vi "Set Value (U32).vi"(8 "error in":errorcluster, 9 "Value":u32, 10 "TPCANParameter":T2, 11 "TPCANHandle in":T1 items=["PCAN_NONEBUS"=0, "PCAN_USBBUS1"=81, "PCAN_USBBUS2"=82, "PCAN_USBBUS3"=83, "PCAN_USBBUS4"=84, "PCAN_USBBUS5"=85, "PCAN_USBBUS6"=86, "PCAN_USBBUS7"=87, "PCAN_USBBUS8"=88, "PCAN_USBBUS9"=1289, "PCAN_USBBUS10"=1290, "PCAN_USBBUS11"=1291, "PCAN_USBBUS12"=1292, "PCAN_USBBUS13"=1293, "PCAN_USBBUS14"=1294, "PCAN_USBBUS15"=1295, "PCAN_USBBUS16"=1296]) -> (0 "error out":errorcluster, 3 "TPCANHandle out":T1 items=["PCAN_NONEBUS"=0, "PCAN_USBBUS1"=81, "PCAN_USBBUS2"=82, "PCAN_USBBUS3"=83, "PCAN_USBBUS4"=84, "PCAN_USBBUS5"=85, "PCAN_USBBUS6"=86, "PCAN_USBBUS7"=87, "PCAN_USBBUS8"=88, "PCAN_USBBUS9"=1289, "PCAN_USBBUS10"=1290, "PCAN_USBBUS11"=1291, "PCAN_USBBUS12"=1292, "PCAN_USBBUS13"=1293, "PCAN_USBBUS14"=1294, "PCAN_USBBUS15"=1295, "PCAN_USBBUS16"=1296], 5 "TPCANStatus":u32)   [LabVIEW 2020, in "PCANBasic.lvlib"]
uses:
  PCANBasic.lvlib
  peak/PCANBasic64.dll
  TPCANParameter.ctl
  TPCANHandle.ctl
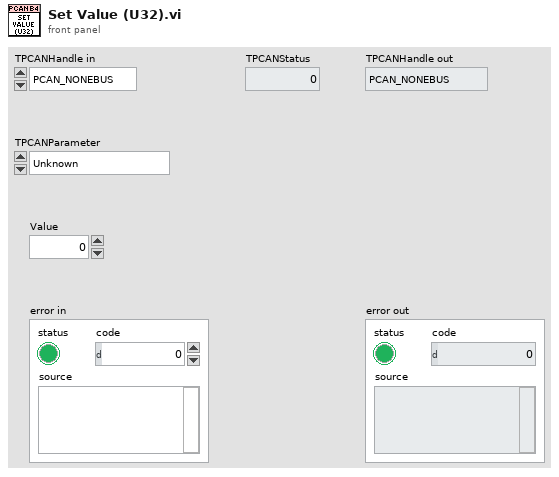
[diagram p1: front panel]
types:
  T1 = typedef "PCANBasic.lvlib/TPCANHandle.ctl" = u16
  T2 = typedef "PCANBasic.lvlib/TPCANParameter.ctl" = enum8{"Unknown", "PCAN_DEVICE_ID", "PCAN_5VOLTS_POWER", "PCAN_RECEIVE_EVENT", "PCAN_MESSAGE_FILTER", "PCAN_API_VERSION", "PCAN_CHANNEL_VERSION", "PCAN_BUSOFF_AUTORESET", "PCAN_LISTEN_ONLY", "PCAN_LOG_LOCATION", "PCAN_LOG_STATUS", "PCAN_LOG_CONFIGURE", "PCAN_LOG_TEXT", "PCAN_CHANNEL_CONDITION", "PCAN_HARDWARE_NAME", "PCAN_RECEIVE_STATUS", "PCAN_CONTROLLER_NUMBER", "PCAN_TRACE_LOCATION", "PCAN_TRACE_STATUS", "PCAN_TRACE_SIZE", "PCAN_TRACE_CONFIGURE", "PCAN_CHANNEL_IDENTIFYING", "PCAN_CHANNEL_FEATURES", "PCAN_BITRATE_ADAPTING", "PCAN_BITRATE_INFO", "PCAN_BITRATE_INFO_FD", "PCAN_BUSSPEED_NOMINAL", "PCAN_BUSSPEED_DATA", "PCAN_IP_ADDRESS", "PCAN_LAN_SERVICE_STATUS", "PCAN_ALLOW_STATUS_FRAMES", "PCAN_ALLOW_RTR_FRAMES", "PCAN_ALLOW_ERROR_FRAMES", "PCAN_INTERFRAME_DELAY", "PCAN_ACCEPTANCE_FILTER_11BIT", "PCAN_ACCEPTANCE_FILTER_29BIT", "PCAN_IO_DIGITAL_CONFIGURATION", "PCAN_IO_DIGITAL_VALUE", "PCAN_IO_DIGITAL_SET", "PCAN_IO_DIGITAL_CLEAR", "PCAN_IO_ANALOG_VALUE", "PCAN_FIRMWARE_VERSION", "PCAN_ATTACHED_CHANNELS_COUNT", "PCAN_ATTACHED_CHANNELS", "PCAN_ALLOW_ECHO_FRAMES", "PCAN_DEVICE_PART_NUMBER", "PCAN_HARD_RESET_STATUS", "PCAN_LAN_CHANNEL_DIRECTION", "PCAN_DEVICE_GUID"}
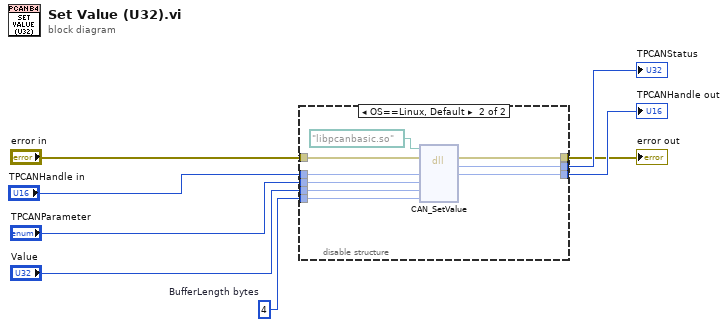
[diagram p0: block diagram]
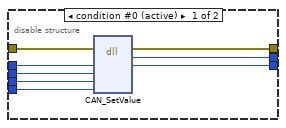
[diagram p2: hidden frame]
diagram:
  w1 = u32 4  # BufferLength bytes
  n1 = disable-structure shown="OS==Linux, Default" {
    disable-tunnel: "TPCANHandle in" -> [w16 w25]
    disable-tunnel: "error in" -> [w15 w24]
    disable-tunnel: [w14 w23] -> w4
    disable-tunnel: "TPCANParameter" -> [w13 w22]
    disable-tunnel: [w12 w21] -> w6
    disable-tunnel: "Value" -> [w11 w20]
    disable-tunnel: [w10 w19] -> w8
    disable-tunnel: w1 -> [w9 w17]
    frame condition #0 (active) {
      n2 = dll-call lib="D:/git/PCAN-Basic-LabVIEW/source/peak/PCANBasic*.dll" fn="CAN_SetValue"(error in=w15, "Channel"=w16, "TPCANParameter"=w13, "Buffer"=w11, "BufferLength"=w9) -> (error out=w14:errorcluster, "TPCANStatus"=w12:u32, "Channel"=w10:u16)  [unwired: 5 in, 1 out]
    }
    frame condition #1 {
      n3 = dll-call lib="libpcanbasic.so" fn="CAN_SetValue"(path in=path "libpcanbasic.so", error in=w24, "Channel"=w25, "TPCANParameter"=w22, "Buffer"=w20, "BufferLength"=w17) -> (error out=w23:errorcluster, "TPCANStatus"=w21:u32, "Channel"=w19:u16)  [unwired: 4 in, 1 out]
    }
  }
  "TPCANHandle out" <- w8
  "TPCANStatus" <- w6
  "error out" <- w4
